vi "W4Q2.vi"() -> ()   [LabVIEW 2021]
panel:
  out "Waveform Graph":dynamicdata(graph)
  in  "f":dbl
  in  "Amp":dbl
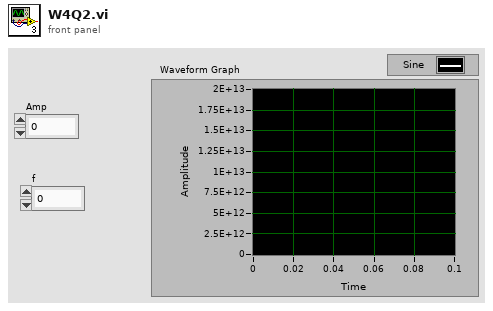
[diagram p1: front panel]
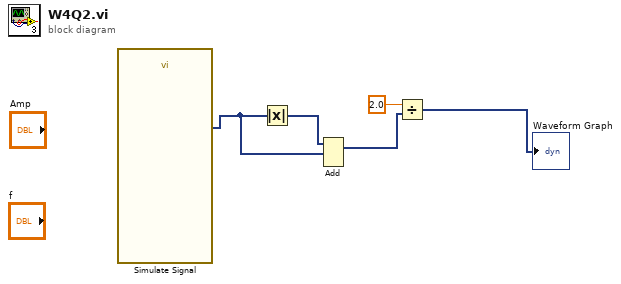
[diagram p0: block diagram]
diagram:
  n1 = call "Simulate Signal"() -> ("Sine"=w3:dynamicdata)  [unwired: 14 in, 1 out]
  n2 = Absolute Value(x=w3) -> (abs(x)=w4:dynamicdata)
  n3 = Add(1:w3, 2:w4) -> (0:w2:dynamicdata)  [unwired: 1 in, 1 out]
  n4 = Divide(x=2.0, y=w2) -> (x/y=→"Waveform Graph":dynamicdata)
